vi "Scan_Check.vi"(6 "SR830状态":bool, 7 "Error In":errorcluster caption="错误输入", 8 "储存路径":path, 9 "字符串参数":T1, 10 "数值参数":T2) -> (0 "Error Out":errorcluster caption="错误输出", 2 "扫描开始时间":dbl, 3 "检查结果":bool)   [LabVIEW 2020]
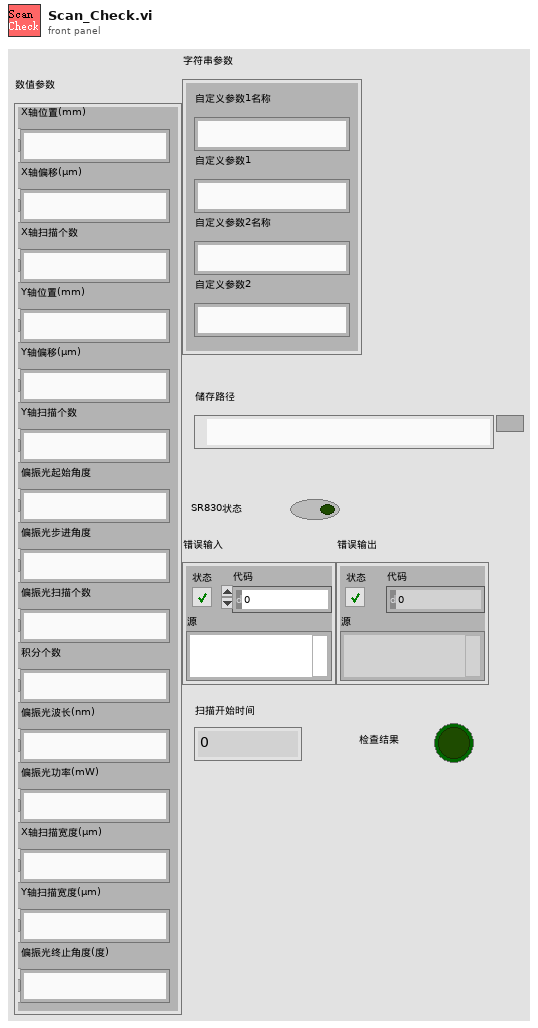
[diagram p1: front panel]
types:
  T1 = cluster{"自定义参数1名称":string, "自定义参数1":string, "自定义参数2名称":string, "自定义参数2":string}
  T2 = cluster{"X轴位置(mm)":dbl, "X轴偏移(μm)":dbl, "X轴扫描个数":dbl, "Y轴位置(mm)":dbl, "Y轴偏移(μm)":dbl, "Y轴扫描个数":dbl, "偏振光起始角度":dbl, "偏振光步进角度":dbl, "偏振光扫描个数":dbl, "积分个数":dbl, "偏振光波长(nm)":dbl, "偏振光功率(mW)":dbl, "X轴扫描宽度(μm)":dbl, "Y轴扫描宽度(μm)":dbl, "偏振光终止角度(度)":dbl}
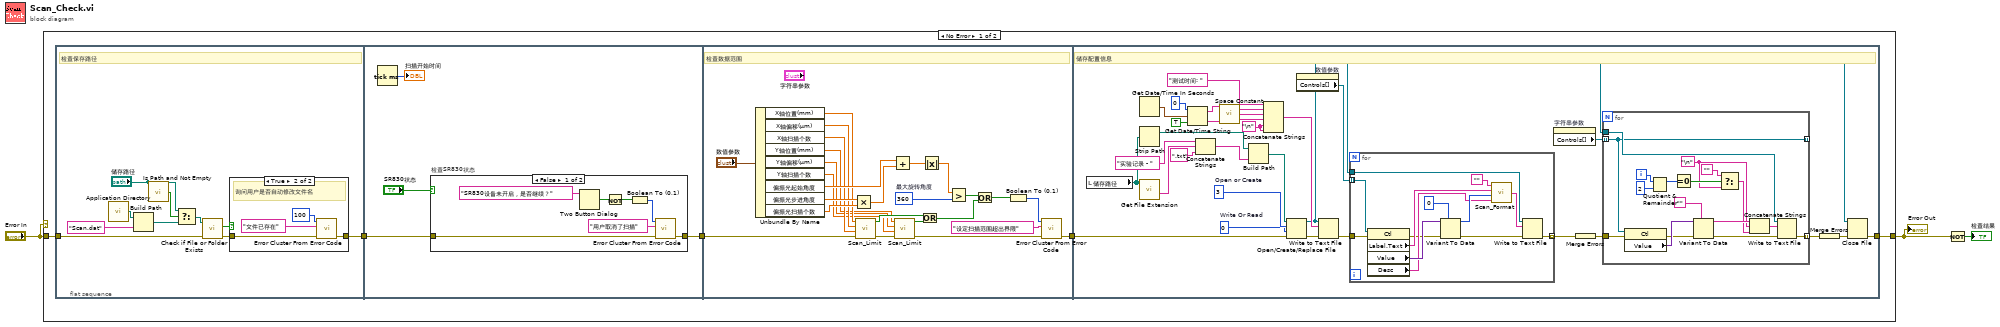
[diagram p0: block diagram]
diagram:
  n1 = case shown="No Error" "Error In" {
    selector: "Error In" -> [_ w120]
    tunnel: [w8 w120] -> w1
    tunnel: "Error In" -> [w6 _]
    frame No Error {
      n2 = flat-sequence {
        tunnel: [w10] -> w4
        tunnel: w6 -> [w9]
        tunnel: [w25] -> w5
        tunnel: w4 -> [w24]
        tunnel: [w46] -> w7
        tunnel: w5 -> [w60]
        tunnel: w7 -> [w87]
        tunnel: [w86] -> w8
        frame #0 {
          # "检查保存路径"
          n3 = call <vilib>:"Application Directory.vi"() -> ("Application Directory"=w14:path)
          n4 = Build Path(base path=w14, name or relative path="Scan.dat") -> (appended path=w12:path)
          n5 = call <vilib>:"Is Path and Not Empty.vi"("path"="储存路径") -> ("Is Path and Not Empty?"=w16:bool)  [unwired: 4 in]
          n6 = Select(t="储存路径", s=w16, f=w12) -> (s? t:f=w11:path)
          n7 = call <vilib>:"Check if File or Folder Exists.vi"("error in (no error)"=w9, "path"=w11) -> ("error out"=w18:errorcluster, "file or folder exists?"=w17:bool)  [unwired: 7 in, 1 out]
          n8 = case shown="True" w17 {
            tunnel: w18 -> [w19 w23]
            tunnel: [w19 w22] -> w10
            frame False {
              # "不做处理"
            }
            frame True {
              # "询问用户是否自动修改文件名"
              n9 = call <vilib>:"Error Cluster From Error Code.vi"("error in (no error)"=w23, "error message (\"\")"="文件已存在", "error code (0)"=100) -> ("error out"=w22:errorcluster)  [unwired: 6 in]
            }
          }
        }
        frame #1 {
          n10 = Tick Count (ms)() -> (millisecond timer value=→"扫描开始时间":u32)
          n11 = case "检查SR830状态" shown="False" "SR830状态" {
            tunnel: w24 -> [w28 w35]
            tunnel: [w29 w35] -> w25
            frame False {
              n12 = Two Button Dialog(message="SR830设备未开启，是否继续？") -> (T button?=w33:bool)  [unwired: 2 in]
              n13 = Not(x=w33) -> (.not. x?=w32:bool)
              n14 = Boolean To (0,1)(Boolean=w32) -> (0, 1=w31:i16)
              n15 = call <vilib>:"Error Cluster From Error Code.vi"("error in (no error)"=w28, "error message (\"\")"="用户取消了扫描", "error code (0)"=w31) -> ("error out"=w29:errorcluster)  [unwired: 6 in]
            }
            frame True {
            }
          }
        }
        frame #2 {
          w53 = 360  # 最大旋转角度
          # "检查数据范围"
          n16 = Unbundle By Name("数值参数") -> ("X轴位置(mm)"=w42:dbl, "X轴偏移(μm)"=w41:dbl, "X轴扫描个数"=w40:dbl, "Y轴位置(mm)"=w39:dbl, "Y轴偏移(μm)"=w38:dbl, "Y轴扫描个数"=w37:dbl, "偏振光起始角度"=w43:dbl, "偏振光步进角度"=w45:dbl, "偏振光扫描个数"=w44:dbl)
          n17 = Multiply(x=w45, y=w44) -> (x*y=w56:dbl)
          n18 = call "Scan_Limit.vi"("Error In"=w60, "扫描个数"=w40, "扫描间隔(μm)"=w41, "当前值(mm)"=w42) -> ("Error Out"=w59:errorcluster, "超出范围"=w58:bool)  [unwired: 6 in]
          n19 = Add(x=w43, y=w56) -> (x+y=w55:dbl)
          n20 = call "Scan_Limit.vi"("Error In"=w59, "扫描个数"=w37, "扫描间隔(μm)"=w38, "当前值(mm)"=w39) -> ("Error Out"=w47:errorcluster, "超出范围"=w57:bool)  [unwired: 6 in]
          n21 = Or(x=w58, y=w57) -> (x .or. y?=w52:bool)
          n22 = Absolute Value(x=w55) -> (abs(x)=w54:dbl)
          n23 = Greater?(x=w54, y=w53) -> (0:w51:bool)
          n24 = Or(x=w51, y=w52) -> (x .or. y?=w50:bool)
          n25 = Boolean To (0,1)(Boolean=w50) -> (0, 1=w48:i16)
          n26 = call <vilib>:"Error Cluster From Error Code.vi"("error in (no error)"=w47, "error message (\"\")"="设定扫描范围超出界限", "error code (0)"=w48) -> ("error out"=w46:errorcluster)  [unwired: 6 in]
        }
        frame #3 {
          w65 = "\n"
          w88 = 0  # Write Or Read
          w89 = 3  # Open or Create
          # "储存配置信息"
          n27 = local read "储存路径"() -> (w64:path)
          n28 = Get Date/Time In Seconds() -> (seconds since 1Jan1904=w81:timestamp)
          n29 = Strip Path(path=w64) -> (stripped path=w63:path)  [unwired: 1 out]
          n30 = call <vilib>:"Get File Extension.vi"("file"=w64) -> ("filename without extension"=w62:string)  [unwired: 6 in, 4 out]
          n31 = Get Date/Time String(date format (0)=0, seconds (now)=w81, want seconds? (F)=TRUE) -> (date string=w79:string, time string=w77:string)
          n32 = Concatenate Strings("实验记录 - ", w62, ".txt") -> (w84:string)
          n33 = call <vilib>:"Space Constant.vi"() -> ("String"=w78:string)
          n34 = Build Path(base path=w63, name or relative path=w84) -> (appended path=w85:path)
          n35 = Concatenate Strings("测试时间: ", w79, w78, w77, w65, w65) -> (w74:string)
          n36 = Open/Create/Replace File(file path (use dialog)=w85, error in=w87, operation (0:open)=w89, access (0:read/write)=w88) -> (refnum out=w69:refnum<file>, error out=w73:errorcluster)  [unwired: 2 in, 1 out]
          n37 = property on="数值参数" class="Clust (strict)"() -> ("Controls[]"=w75:refnum<vi>[])  [unwired: 2 in, 2 out]
          n38 = Write to Text File(file (use dialog)=w69, text=w74, error in=w73) -> (error out=w72:errorcluster)  [unwired: 1 in, 2 out]
          n39 = for {
            tunnel: w75 -> [w119] mode=indexing
            tunnel: w69 -> [w111]
            tunnel: w72 -> [w110]
            tunnel: [w107] -> w71 mode=indexing
            n40 = property on="属性节点" class="Ctl"(reference=w119, error in=w110) -> (error out=w109:errorcluster, "Label.Text"=w117:string, "Value"=w116:variant, "Desc"=w113:string)  [unwired: 1 out]
            n41 = Variant To Data(error in=w109, type=0, Variant=w116) -> (data=w114:i32, error out=w108:errorcluster)
            n42 = call "Scan_Format.vi"("字符串格式(%.6f)"=w113, "要转化的数字"=w114, "数字标题"=w117, "原始字符串"="") -> ("输出转换结果"=w112:string)
            n43 = Write to Text File(file (use dialog)=w111, text=w112, error in=w108) -> (error out=w107:errorcluster)  [unwired: 1 in, 2 out]
          }
          n44 = property on="字符串参数" class="Clust (strict)"() -> ("Controls[]"=w70:refnum<vi>[])  [unwired: 2 in, 2 out]
          n45 = Merge Errors(w71) -> (w68:errorcluster)
          n46 = for {
            tunnel: [w100] -> _ mode=indexing
            tunnel: w69 -> [w105]
            tunnel: w68 -> [w104]
            tunnel: [w101] -> w67 mode=indexing
            tunnel: w70 -> [w100] mode=indexing
            i -> [w97]
            w90 = "\n"
            n47 = property on="属性节点" class="Ctl"(reference=w100, error in=w104) -> (error out=w103:errorcluster, "Value"=w106:variant)  [unwired: 1 out]
            n48 = Quotient & Remainder(x=w97, y=2) -> (x-y*floor(x/y)=w95:i32)  [unwired: 1 out]
            n49 = Equal To 0?(x=w95) -> (x = 0?=w94:bool)
            n50 = Variant To Data(error in=w103, type="", Variant=w106) -> (data=w93:string, error out=w102:errorcluster)
            n51 = Select(t="", s=w94, f=w90) -> (s? t:f=w91:string)
            n52 = Concatenate Strings(w93, w90, w91) -> (w98:string)
            n53 = Write to Text File(file (use dialog)=w105, text=w98, error in=w102) -> (error out=w101:errorcluster)  [unwired: 1 in, 2 out]
          }
          n54 = Merge Errors(w67) -> (w66:errorcluster)
          n55 = Close File(refnum=w69, error in=w66) -> (error out=w86:errorcluster)  [unwired: 1 out]
        }
      }
    }
    frame Error {
    }
  }
  "Error Out" <- w1
  n56 = Not(x=w1) -> (.not. x?=→"检查结果":bool)
